vi "HEWH Set C1 or C2.vi"(8 "Error In":errorcluster, 11 "Full Cutout?":bool) -> (0 "Error Out":errorcluster, 3 "Current Cond Out":T1)   [LabVIEW 2016]
uses:
  Type Definitions/HEWH Special Condition Check.ctl
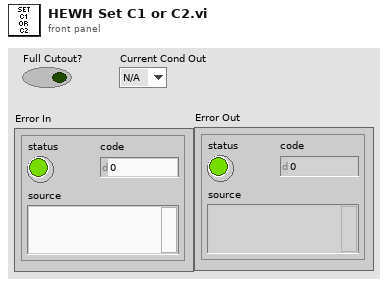
[diagram p1: front panel]
types:
  T1 = typedef "HEWH Special Condition Check.ctl" = enum16{"N/A", "C1", "C2", "Reset/Fail", "Skip Draw Sequence"}
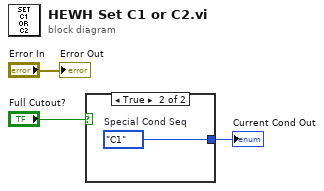
[diagram p0: block diagram]
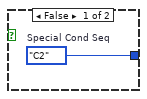
[diagram p2: hidden frame]
diagram:
  n1 = case shown="True" "Full Cutout?" {
    tunnel: [w4 w5] -> w3
    frame False {
      w4 = HEWH_Special_Condition_Check."C2"  # Special Cond Seq
    }
    frame True {
      w5 = HEWH_Special_Condition_Check."C1"  # Special Cond Seq
    }
  }
  "Current Cond Out" <- w3
  "Error Out" <- "Error In"
